vi "S1500_S7Com_SQLtoPLC_1500.vi"(11 "Variablen IN":T1={"DB"=0, "Adresse"=0, "Länge"=0, "Typ"=enum."BYTE", "Enum"=enum."WRITE"}) -> (3 "RW_CMD":T4={"Read Length"=0, "Data Block #"=0, "S7_Add_Area"=0, "Start Address"=0, "S7_Transport_Size"=1, "S7_Function"=0, "IP-Address"=""} {"S7_Function" items=["Read"=4, "Write"=5]; "S7_Transport_Size" items=["BIT"=1, "BYTE"=2, "CHAR"=3, "WORD"=4, "INT"=5, "DWORD"=6, "DINT"=7, "REAL"=8]; "S7_Add_Area" items=["P Area"=128, "I Area"=129, "O Area"=130, "M Area"=131, "DB Area"=132, "Counter"=40, "Timer"=41]})   [LabVIEW 2018]
uses:
  S1500_S7Com_RW_CMD.ctl
  S1500_S7Com_Address_Area.ctl
  S1500_S7Com_Start_Add.ctl
  S1500_S7Com_Transport_Size.ctl
  S1500_S7Com_Function.ctl
  S1500_ENUM Typ.ctl
  S1500_S7Com_DATATypes.ctl
  S1500_S7Com_RW.ctl
  S7Com_Source_inkl_IP/S7Com_Address_Area.ctl
  S7Com_Source_inkl_IP/S7Com_DATATypes.ctl
  S7Com_Source_inkl_IP/S7Com_Function.ctl
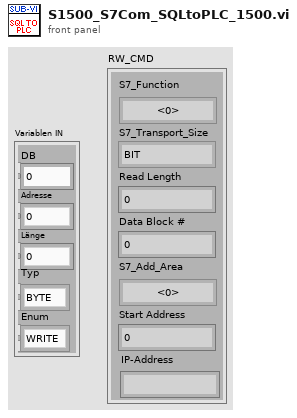
[diagram p1: front panel]
types:
  T1 = typedef "S1500_ENUM Typ.ctl" = cluster{"DB":u32, "Adresse":u32, "Länge":u32, "Typ":T2, "Enum":T3}
  T2 = typedef "S1500_S7Com_DATATypes.ctl" = enum16{"", "BIT", "BYTE", "CHAR", "WORD", "INT", "DWORD", "DINT", "REAL", "STRING"}
  T3 = typedef "S1500_S7Com_RW.ctl" = enum16{"WRITE", "READ"}
  T4 = typedef "S1500_S7Com_RW_CMD.ctl" = cluster{"Read Length":u16, "Data Block #":u16, "S7_Add_Area":T5, "Start Address":T6, "S7_Transport_Size":T7, "S7_Function":T8, "IP-Address":string}
  T5 = typedef "S1500_S7Com_Address_Area.ctl" = u8
  T6 = typedef "S1500_S7Com_Start_Add.ctl" = u16
  T7 = typedef "S1500_S7Com_Transport_Size.ctl" = u8
  T8 = typedef "S1500_S7Com_Function.ctl" = u8
  T9 = typedef "S7Com_DATATypes.ctl" = enum16{"", "BIT", "BYTE", "CHAR", "WORD", "INT", "DWORD", "DINT", "REAL"}
  T10 = typedef "S7Com_Address_Area.ctl" = u8
  T11 = typedef "S7Com_Function.ctl" = u8
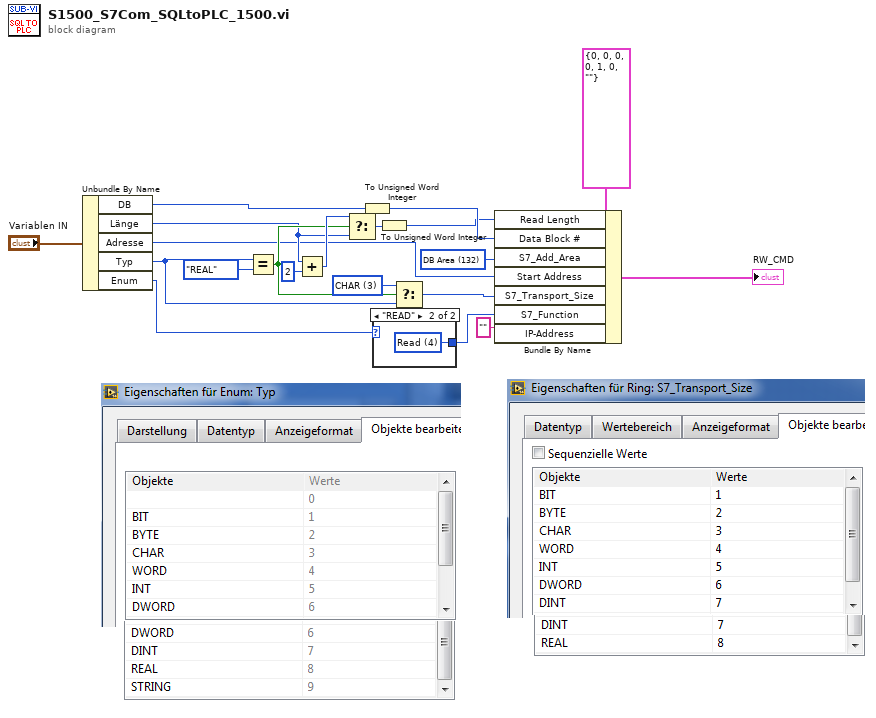
[diagram p0: block diagram]
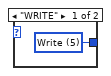
[diagram p2: hidden frame]
diagram:
  w3 = T7 3 items=["BIT"=1, "BYTE"=2, "CHAR"=3, "WORD"=4, "INT"=5, "DWORD"=6, "DINT"=7, "REAL"=8] ("S7_Transport_Size")
  w20 = T10 132 items=["P Area"=128, "I Area"=129, "O Area"=130, "M Area"=131, "DB Area"=132, "Counter"=40, "Timer"=41] ("S7_Add_Area")
  n1 = Unbundle By Name("Variablen IN") -> ("DB"=w16:u32, "Länge"=w6:u32, "Adresse"=w1:u32, "Typ"=w4:T2, "Enum"=w18:T3)
  n2 = Equal?(x=w4, y=S7Com_DATATypes."REAL") -> (x = y?=w10:bool)
  n3 = Add(x=w6, y=u32 2) -> (x+y=w11:u32)
  n4 = Select(t=w11, s=w10, f=w6) -> (s? t:f=w9:u32)
  n5 = To Unsigned Word Integer(number=w16) -> (unsigned 16bit integer=w15:u16)
  n6 = case shown="\"READ\"" w18 {
    tunnel: [w21 w22] -> w17
    frame "WRITE" {
      w21 = T11 5 items=["Read"=4, "Write"=5] ("S7_Function")
    }
    frame "READ" {
      w22 = T11 4 items=["Read"=4, "Write"=5] ("S7_Function")
    }
  }
  n7 = To Unsigned Word Integer(number=w9) -> (unsigned 16bit integer=w5:u16)
  n8 = Select(t=w3, s=w10, f=w4) -> (s? t:f=w2:u16)
  n9 = Bundle By Name(cluster=T4 {"Read Length"=0, "Data Block #"=0, "S7_Add_Area"=0, "Start Address"=0, "S7_Transport_Size"=1, "S7_Function"=0, "IP-Address"=""} ("RW_CMD"), "Read Length"=w5, "Data Block #"=w15, "S7_Add_Area"=w20, "Start Address"=w1, "S7_Transport_Size"=w2, "S7_Function"=w17, "IP-Address"="") -> (→"RW_CMD":T4)
